vi "IndoorData_Init.vi"(0 "reference in":refnum<class "IndoorData.lvclass"> caption="This control should only be used when\na sub class is inheriting this class", 5 "error in (no error)":errorcluster) -> (14 "reference out":refnum<class "IndoorData.lvclass"> caption="This indicator should only be used when\na sub class is inheriting this class", 19 "error out":errorcluster)   [LabVIEW 2014, in "IndoorData.lvclass"]
uses:
  IndoorData.lvclass
  DebugData.ctl
  ActualValues.ctl
  BufferedReadings.ctl
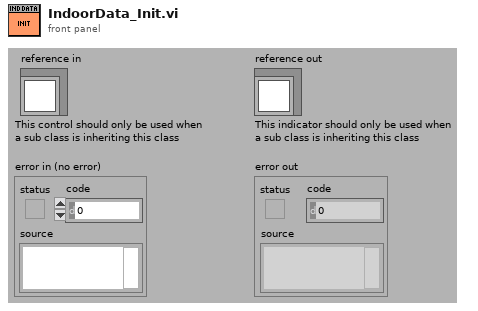
[diagram p1: front panel]
types:
  T1 = typedef "IndoorData.lvclass/BufferedReadings.ctl" = cluster{"Time":dbl[], "Temp":dbl[], "RH":dbl[]}
  T2 = typedef "IndoorData.lvclass/ActualValues.ctl" = cluster{"Time":dbl, "Temp":dbl, "RH":dbl}
  T3 = typedef "IndoorData.lvclass/DebugData.ctl" = cluster{"Rev":string, "Location":string, "LoopIdx":i32, "PiCoreTemp":dbl, "Error":errorcluster}
  T4 = typedef "IndoorData.lvclass/ObjectAttributes.ctl" = cluster{"DebugData":T3, "Actual":T2, "BufferedReadings":T1, "AVGReadings":T1, "DataFolder":path, "FirstLog?":bool}
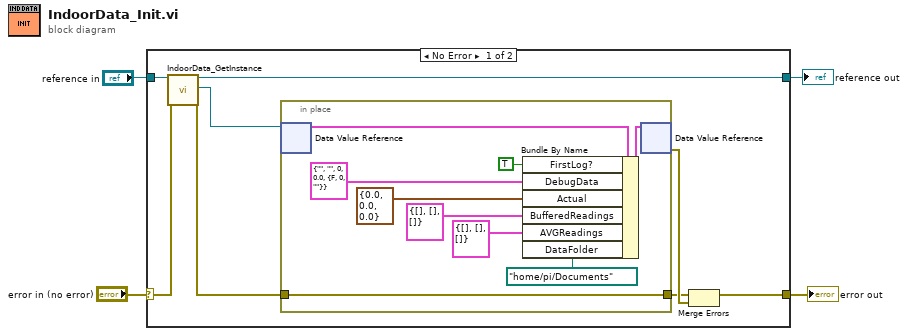
[diagram p0: block diagram]
diagram:
  n1 = case shown="No Error" "error in (no error)" {
    selector: "error in (no error)" -> [w10 w23]
    tunnel: [w11 w23] -> w3
    tunnel: "reference in" -> [w9 w22]
    tunnel: [w8 w22] -> w1
    frame No Error {
      n2 = call "IndoorData_GetInstance.vi"("reference in"=w9, "error in (no error)"=w10) -> ("reference out"=w8:refnum<class "IndoorData.lvclass">, "DVRRefOut"=w7:refnum<data-value>, "error out"=w5:errorcluster)  [unwired: 13 in, 2 out]
      n3 = in-place {
        in-place-border: w5 -> [w19]
        in-place-border: [w19] -> w6
        n4 = in-place-dvr #1(w7) -> (w20:T4)  [unwired: 1 out]
        n5 = Bundle By Name(cluster=w20, "FirstLog?"=TRUE ("Reboot?"), "DebugData"=T3 {"Rev"="", "Location"="", "LoopIdx"=0, "PiCoreTemp"=0.0, "Error"={"status"=FALSE, "code"=0, "source"=""}}, "Actual"=T2 {"Time"=0.0, "Temp"=0.0, "RH"=0.0}, "BufferedReadings"=T1 {"Time"=[], "Temp"=[], "RH"=[]}, "AVGReadings"=T1 {"Time"=[], "Temp"=[], "RH"=[]}, "DataFolder"=path "/home/pi/Documents") -> (w21:T4)
        n6 = in-place-dvr #1(w21) -> (w12:errorcluster)  [unwired: 1 out]
      }
      n7 = Merge Errors(w6, w12) -> (w11:errorcluster)
    }
    frame Error {
    }
  }
  "error out" <- w3
  "reference out" <- w1
